vi "Configuration Window.vi"(8 "error in (no error)":errorcluster, 11 "Inst.MOTOR in":refnum<class "Inst.MOTOR.lvclass">) -> (0 "error out":errorcluster, 3 "Inst.MOTOR out":refnum<class "Inst.MOTOR.lvclass">)   [LabVIEW 2019, in "Inst.MOTOR.lvclass"]
uses:
  Inst.MOTOR.lvclass
  Inst.MOTOR.lvclass/Inst.MOTOR.ctl
  <userlib>/LevyLab/Instrument Framework/Instrument Types/VSource/Instrument.VSource.lvclass
panel:
  in  "Termination Character":u8=10 format="%.0x"
  in  "Address":refnum<visa-resource-name>
  in  "flow control":u16(ring) items=["None"=0, "XON/XOFF"=1, "RTS/CTS"=2, "DTR/DSR"=4]
  in  "stop bits":u16(ring)=10 items=["1.0"=10, "1.5"=15, "2.0"=20]
  in  "baud rate":u32(ring)=9600 items=["75"=75, "110"=110, "134"=134, "150"=150, "300"=300, "600"=600, "1200"=1200, "1800"=1800, "2400"=2400, "4800"=4800, "7200"=7200, "9600"=9600, "14400"=14400, "19200"=19200, "28800"=28800, "38400"=38400, "56000"=56000, "57600"=57600, "115200"=115200, "128000"=128000, "230400"=230400]
  in  "parity":enum16{"None", "Odd", "Even", "Mark", "Space"}(ring)
  in  "data bits":u16=8 min=5 max=8 step=1
  in  "Cancel":bool
  in  "OK":bool
  # "confirm or make changes:"
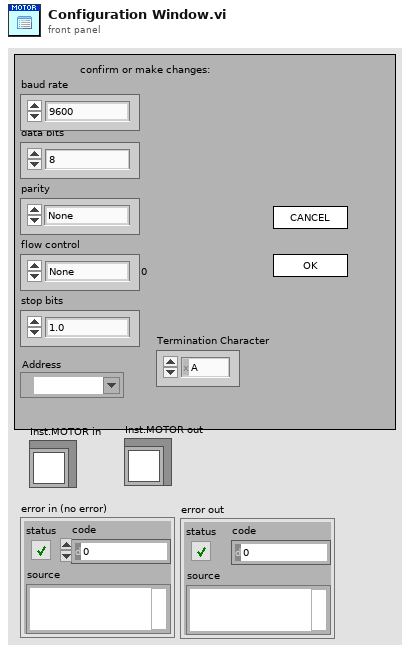
[diagram p1: front panel]
types:
  T1 = enum32{"Invalid", "Standard", "Closed", "Hidden", "Minimized", "Maximized"}
  T2 = enum32{"invalid app kind", "Development System", "Run Time System", "Student Edition", "Embedded LabVIEW", "Evaluation", "Custom"}
  T3 = typedef "Inst.MOTOR.lvclass/Inst.MOTOR.Configuration--Cluster.ctl" = cluster{"baud rate":u32, "data bits":u16, "parity":enum16{"None", "Odd", "Even", "Mark", "Space"}, "stop bits":u16, "flow control":u16, "Read Count":u32, "Address":refnum<visa-resource-name>, "Termination Character":u8}
  T4 = cluster{"Core":cluster{"Current VI Reference":refnum<vi>, "Close Panel on Exit?":bool}, "Configuration":T3}
  T5 = cluster{"Current VI Reference":refnum<vi>, "Close Panel on Exit?":bool}
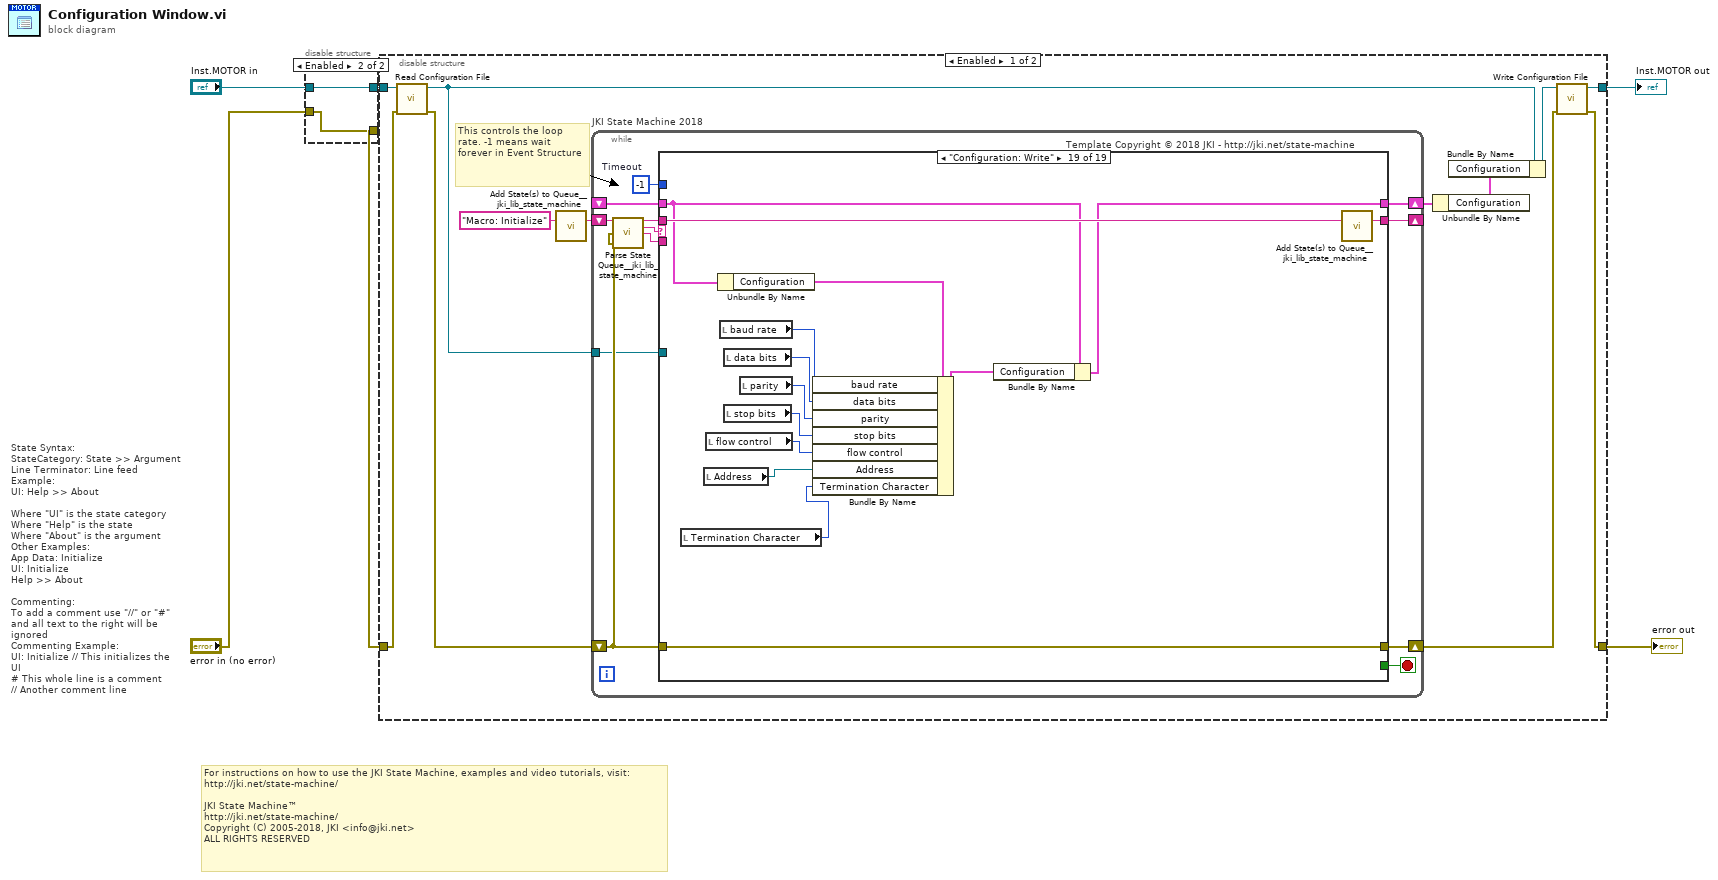
[diagram p0: block diagram]
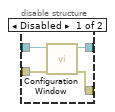
[diagram p2: hidden frame]
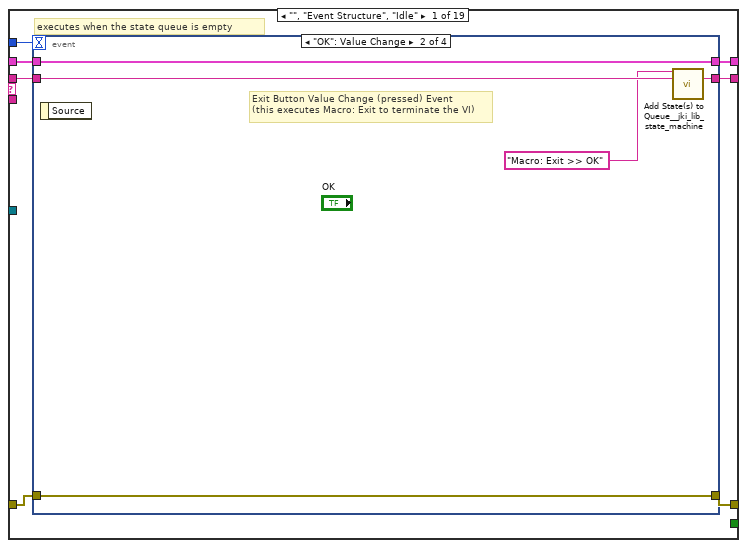
[diagram p3: hidden frame]
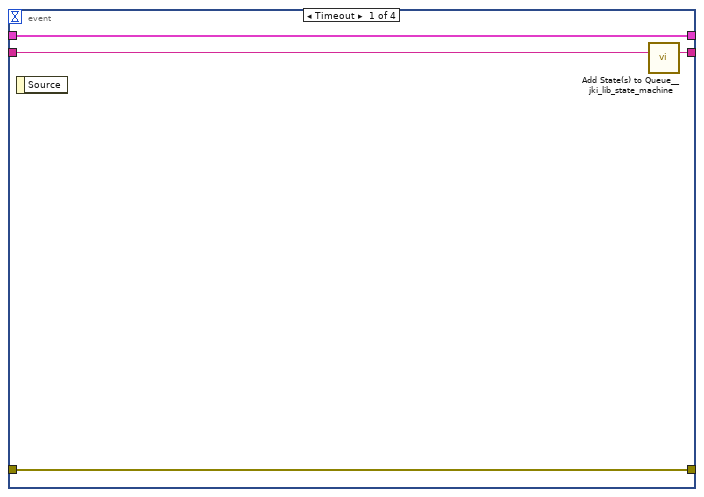
[diagram p4: hidden frame]
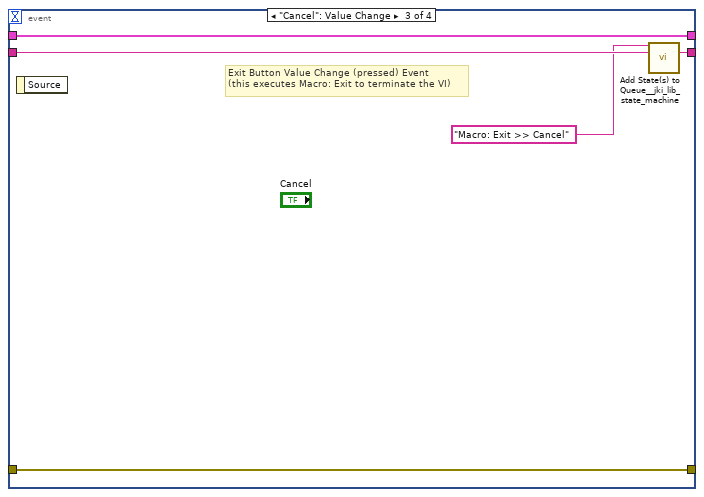
[diagram p5: hidden frame]
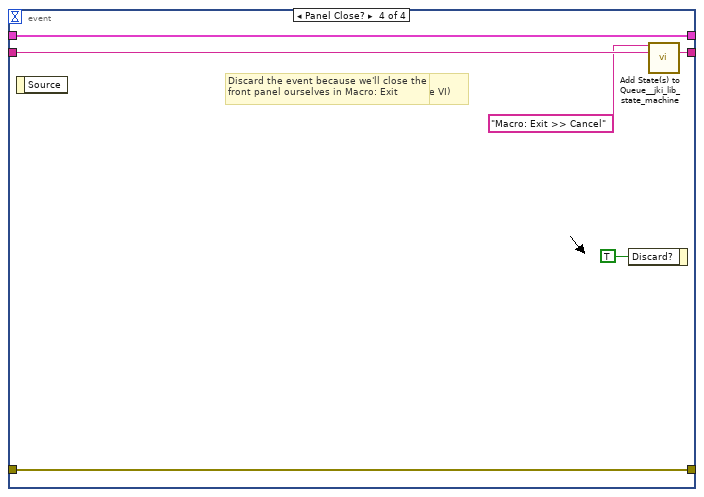
[diagram p6: hidden frame]
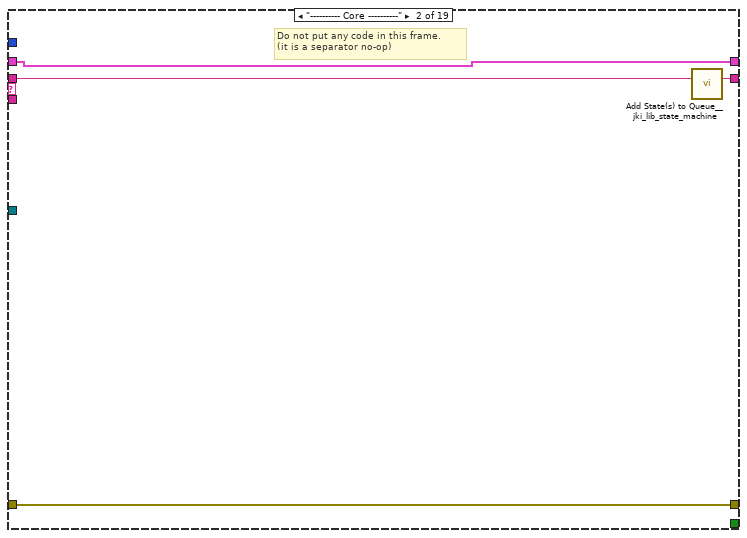
[diagram p7: hidden frame]
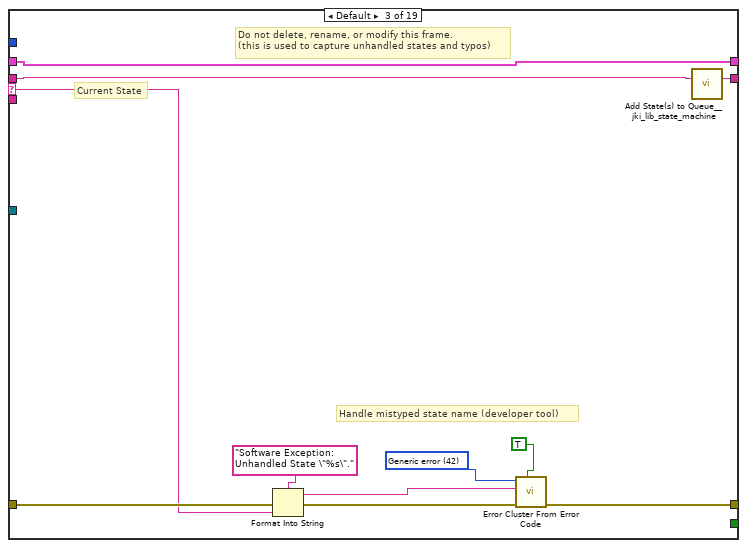
[diagram p8: hidden frame]
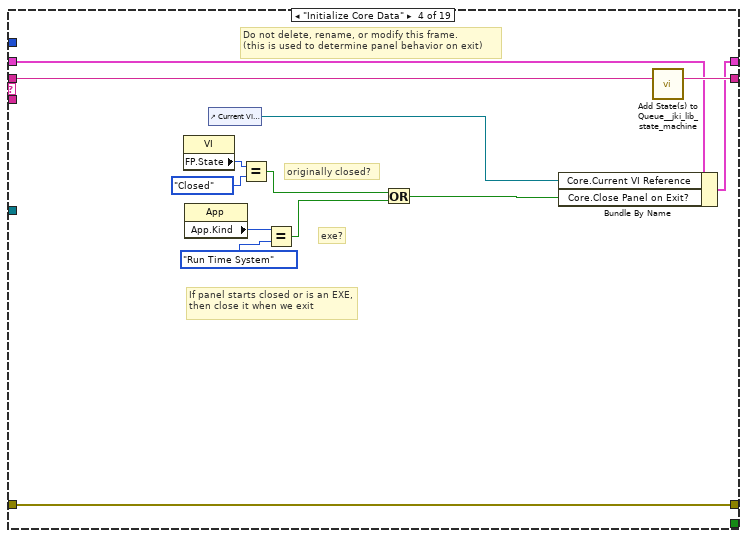
[diagram p9: hidden frame]
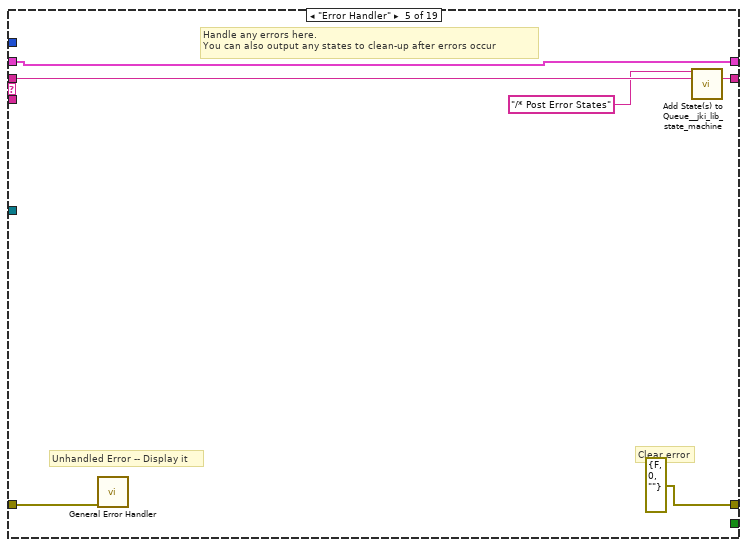
[diagram p10: hidden frame]
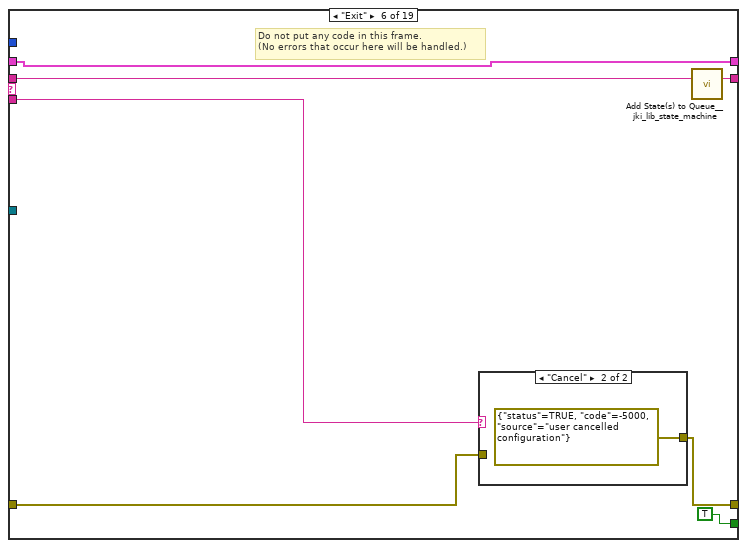
[diagram p11: hidden frame]
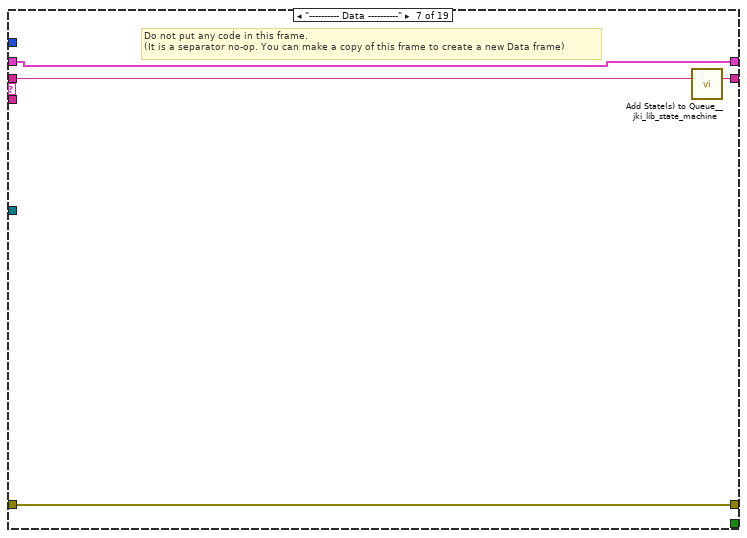
[diagram p13: hidden frame]
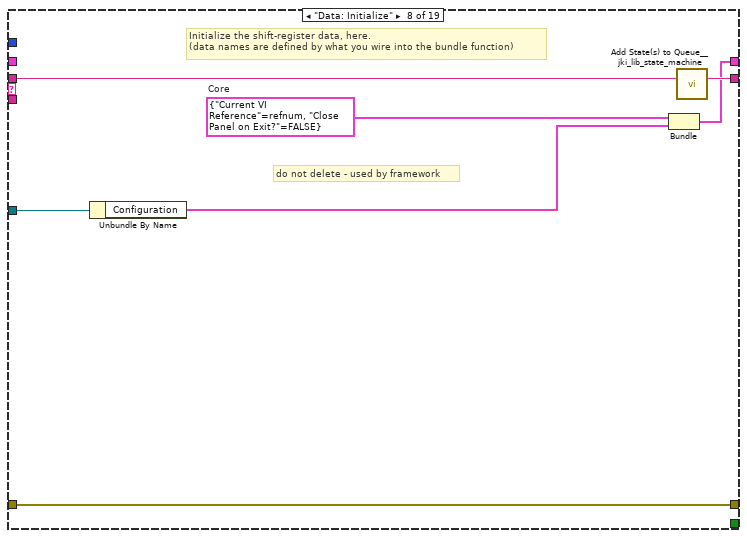
[diagram p14: hidden frame]
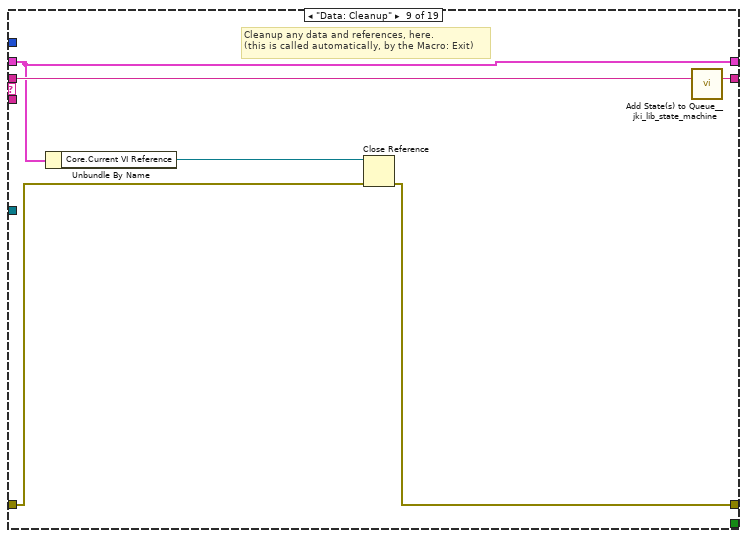
[diagram p15: hidden frame]
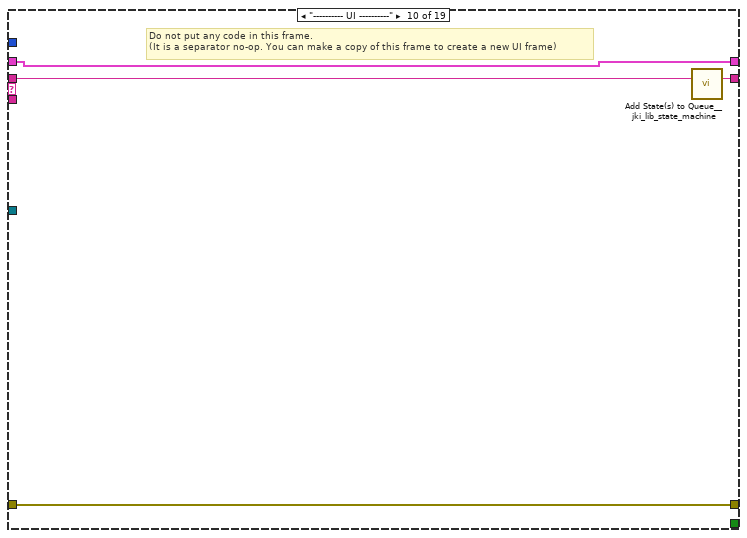
[diagram p16: hidden frame]
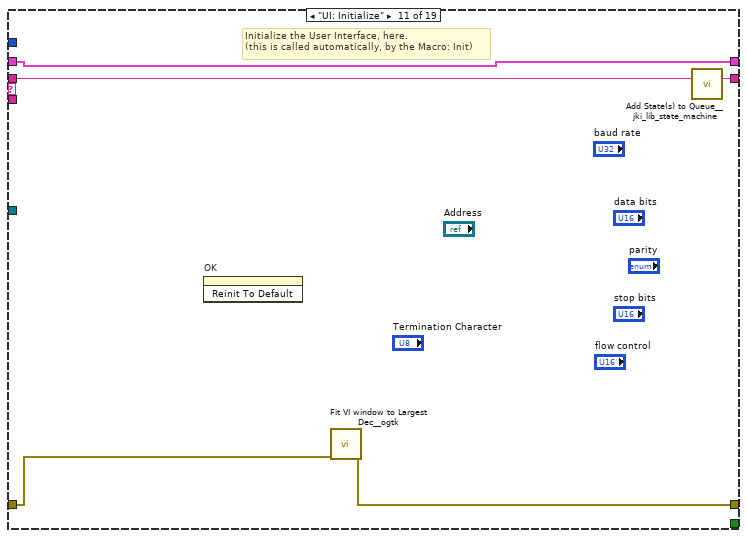
[diagram p17: hidden frame]
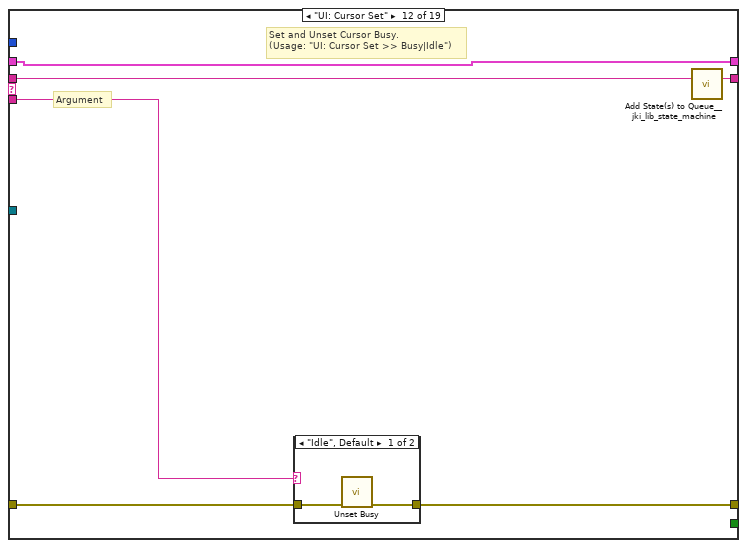
[diagram p18: hidden frame]
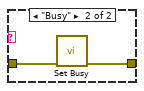
[diagram p19: hidden frame]
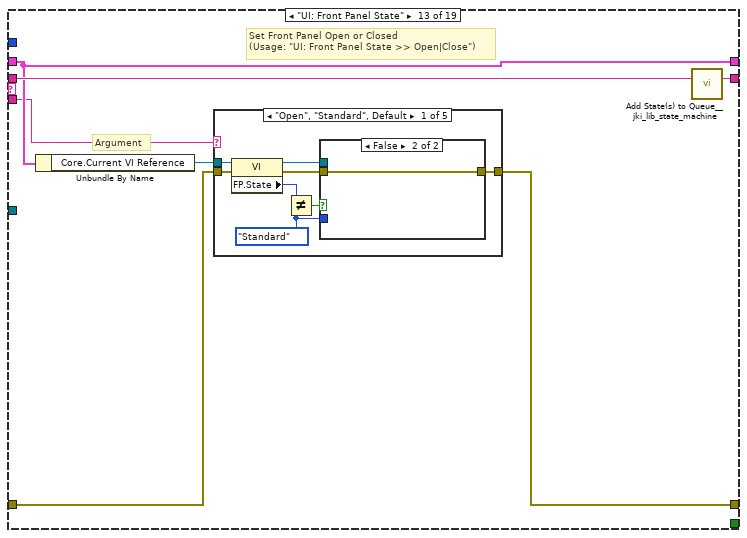
[diagram p20: hidden frame]
diagram:
  # "For instructions on how to use the JKI State Machine, examples and video tutorials, visit:\nhttp://jki.net/state-machine/\n\nJKI State Machine™\nhttp://jki.net/state-machine/\nCopyright (C) 2005-2018, JKI <info@jki.net>\nALL RIGHTS RESERVED"
  # "State Syntax:\nStateCategory: State >> Argument\nLine Terminator: Line feed\nExample:\nUI: Help >> About\n\nWhere \"UI\" is the state category\nWhere \"Help\" is the state\nWhere \"About\" is the argument\nOther Examples:\nApp Data: Initialize\nUI: Initialize\nHelp >> About\n\nCommenting:\nTo add a comment use \"//\" or \"#\" and all text to the right will be ignored\nCommenting Example:\nUI: Initialize // This initializes the UI\n# This whole line is a comment\n// Another comment line"
  n1 = disable-structure shown="Enabled" {
    disable-tunnel: "Inst.MOTOR in" -> [w10 w12]
    disable-tunnel: [w9 w12] -> w3
    disable-tunnel: "error in (no error)" -> [w8 w11]
    disable-tunnel: [w7 w11] -> w1
    frame Disabled {
      n2 = call-parent "Configuration Window.vi"("error in (no error)"=w8, "Instrument"=w10) -> ("error out"=w7:errorcluster, "Instrument out"=w9:refnum<class "Inst.MOTOR.lvclass">)  [unwired: 8 in]
    }
    frame Enabled {
    }
  }
  n3 = disable-structure shown="Enabled" {
    disable-tunnel: [w18 w268] -> w6
    disable-tunnel: [w16 w269] -> w5
    disable-tunnel: w3 -> [w14 w268]
    disable-tunnel: w1 -> [w13 w269]
    frame Enabled {
      # "This controls the loop rate. -1 means wait forever in Event Structure"
      n4 = call-dynamic "Read Configuration File.vi"("error in (no error)"=w13, "Inst.MOTOR in"=w14) -> ("error out"=w15:errorcluster, "Inst.MOTOR out"=w20:refnum<class "Inst.MOTOR.lvclass">)  [unwired: 8 in]
      n5 = call <vilib>:"Add State(s) to Queue__jki_lib_state_machine.vi"("State(s) in (\"\")"="Macro: Initialize") -> ("States Out"=w24:string)  [unwired: 14 in]
      n6 = while "JKI State Machine 2018" {
        shift-right: [w29] -> w22
        shift-left: _ -> [w28]
        shift-right: [w32] -> w17
        shift-left: w15 -> [w26]
        shift-right: [w31] -> _
        shift-left: w24 -> [w33]
        tunnel: w20 -> [w25]
        stop <- w30 stop-if-true
        w27 = -1  # Timeout
        # "Template Copyright © 2018 JKI - http://jki.net/state-machine"
        n7 = call <vilib>:"Parse State Queue__jki_lib_state_machine.vi"("State Queue"=w33, "Error In (no error)"=w26) -> ("Remaining States"=w35:string, "Current State"=w36:string, "Arguments"=w34:string)  [unwired: 11 in]
        n8 = case shown="\"Configuration: Write\"" w36 {
          selector: w36 -> [_ _ w68 _ _ _ _ _ _ _ _ _ _ _ _ _ _ _ _]
          tunnel: w35 -> [w43 w67 w72 w91 w97 w104 w110 w117 w123 w127 w132 w138 w149 w218 w223 w238 w242 w253 w267]
          tunnel: w34 -> [_ _ _ _ _ w100 _ _ _ _ _ w133 w143 _ _ w227 _ _ _]
          tunnel: w28 -> [w41 w64 w70 w84 w94 w102 w107 _ w118 w124 w130 w136 w145 w215 w220 w235 w239 w250 w262]
          tunnel: [w40 w65 w74 w88 errorcluster {"status"=FALSE, "code"=0, "source"=""} ("error out") w98 w108 w113 w119 w125 w128 w134 w146 w216 w221 w236 w240 w251 w265] -> w32
          tunnel: w26 -> [w39 w65 w73 w88 w93 w99 w108 w113 w120 w125 w129 w135 w147 w216 w221 w236 w240 w251 w265]
          tunnel: [w42 w66 w71 w90 w96 w103 w109 w116 w122 w126 w131 w137 w148 w217 w222 w237 w241 w252 w266] -> w31
          tunnel: [_ _ _ _ _ TRUE _ _ _ _ _ _ _ _ _ _ _ _ _] -> w30
          tunnel: [w38 w64 w70 w89 w94 w102 w107 w115 w118 w124 w130 w136 w145 w215 w220 w235 w239 w250 w261] -> w29
          tunnel: w27 -> [w37 _ _ _ _ _ _ _ _ _ _ _ _ _ _ _ _ _ _]
          tunnel: w25 -> [_ _ _ _ _ _ _ w112 _ _ _ _ _ _ _ _ _ _ _]
          frame "", "Event Structure", "Idle" {
            # "executes when the state queue is empty"
            n9 = event shown="[1] \"OK\": Value Change" {
              selector: _ -> [_ _ _ _]
              dyn-events: _ -> [_ _ _ _]
              timeout: w37 -> [_ _ _ _]
              tunnel: w43 -> [w47 w52 w57 w63]
              tunnel: [w46 w51 w56 w62] -> w42
              tunnel: w41 -> [w44 w49 w54 w60]
              tunnel: [w45 w50 w55 w61] -> w40
              tunnel: w39 -> [w45 w50 w55 w61]
              tunnel: [w44 w49 w54 w60] -> w38
              event Timeout {
                n10 = event-data() -> ()  [unwired: 1 in, 1 out]
                n11 = call <vilib>:"Add State(s) to Queue__jki_lib_state_machine.vi"("State(s) in (\"\")"=w47) -> ("States Out"=w46:string)  [unwired: 14 in]
              }
              event "OK": Value Change {
                # "Exit Button Value Change (pressed) Event\n(this executes Macro: Exit to terminate the VI)"
                n12 = event-data() -> ()  [unwired: 1 in, 1 out]
                n13 = call <vilib>:"Add State(s) to Queue__jki_lib_state_machine.vi"("State(s) in Front (\"\")"="Macro: Exit >> OK", "State(s) in (\"\")"=w52) -> ("States Out"=w51:string)  [unwired: 13 in]
              }
              event "Cancel": Value Change {
                # "Exit Button Value Change (pressed) Event\n(this executes Macro: Exit to terminate the VI)"
                n14 = event-data() -> ()  [unwired: 1 in, 1 out]
                n15 = call <vilib>:"Add State(s) to Queue__jki_lib_state_machine.vi"("State(s) in Front (\"\")"="Macro: Exit >> Cancel", "State(s) in (\"\")"=w57) -> ("States Out"=w56:string)  [unwired: 13 in]
              }
              event Panel Close? {
                # "Discard the event because we'll close the front panel ourselves in Macro: Exit"
                # "Close Panel button (pressed) Event\n(this executes Macro: Exit to terminate the VI)"
                n16 = event-data() -> ()  [unwired: 1 in, 1 out]
                n17 = event-data("Discard?"=TRUE) -> ()  [unwired: 1 in, 1 out]
                n18 = call <vilib>:"Add State(s) to Queue__jki_lib_state_machine.vi"("State(s) in Front (\"\")"="Macro: Exit >> Cancel", "State(s) in (\"\")"=w63) -> ("States Out"=w62:string)  [unwired: 13 in]
              }
            }
          }
          frame "---------- Core ----------" {
            # "Do not put any code in this frame.\n(it is a separator no-op)"
            n19 = call <vilib>:"Add State(s) to Queue__jki_lib_state_machine.vi"("State(s) in (\"\")"=w67) -> ("States Out"=w66:string)  [unwired: 14 in]
          }
          frame Default {
            w77 = 42 items=["No error", "Argument error", "Memory is full", "Out of zone", "End of file", "File already open", "Generic file I/O error", "File not found", "File permission error", "Disk is full", "Duplicate path", "Too many files open", "System feature not enabled", "Resource file not found", "Cannot add resource", "Resource not found", "Image not found", "Image memory error", "Pen does not exist", "Config type invalid", "Config token not found", "Config parse error", "Config memory error", "Bad external code format", "Bad external code offset", "External code not present", "Null window", "Destroy window error", "Null menu", "Print aborted", "Bad print record", "Print driver error", "Windows error during printing", "Memory error during printing", "Print dialog error", "Generic print error", "Invalid device refnum", "Device not found", "Device parameter error", "Device unit error", "Cannot open device", "Device call aborted", "Generic error", "Cancelled by user", "Object ID too low", "Object ID too high", "Object not in heap", "Unknown heap", "Unknown object (invalid DefProc)", "Unknown object (DefProc not in table)", "Message out of range", "Invalid (null) method", "Unknown message", "Manager call not supported", "Bad address", "Network operation in progress", "Network operation timed out", "Connection is busy", "Network attribute not supported", "Network error", "Address in use", "System out of memory", "Connection aborted", "Connection refused", "Not connected", "Already connected", "Connection closed", "Initialization error (interapplication manager)", "Bad occurrence", "Wait on unbound occurrence handler", "Occurrence queue overflow", "Datalog type conflict", "Unused", "Unrecognized type (interapplication manager)", "Memory corrupt", "Failed to make temporary DLL", "Old CIN version", "Drag socket not found", "Failed to load drop-object", "Failed to register OLE object", "Failed to release OLE object", "Format specifier type mismatch", "Unknown format specifier", "Too few format specifiers", "Too many format specifiers", "Scan failed", "Newer CIN version", "Error converting to variant", "Runtime menu error", "Password tampered", "Variant attribute not found", "Incompatible variant data type", "Event data is not available", "Event Store is not present", "Occurrence is not found", "Event Queue is not created", "Event info is not available", "Refnum passed is NULL", "Error retrieving Class GUID", "Error retrieving CoClass GUID", "Error retrieving TypeLib GUID.", "Bad built application magic bytes.", "Specific driver is different from the specific driver associated with the Logical Name.", "There is no session opened to the class driver.", "Max Error", "MAX - Error with config objects", "MAX - Error loading configuration", "MAX - Group not supported"]
            # "Current State"
            # "Do not delete, rename, or modify this frame.\n(this is used to capture unhandled states and typos)"
            # "Handle mistyped state name (developer tool)"
            n20 = Format Into String(format string="Software Exception: Unhandled State \"%s\"." ("message"), error in=w73, w68) -> (resulting string=w76:string, error out=w75:errorcluster)  [unwired: 1 in]
            n21 = call <vilib>:"Error Cluster From Error Code.vi"("show call chain? (False)"=TRUE, "error in (no error)"=w75, "error message (\"\")"=w76, "error code (0)"=w77) -> ("error out"=w74:errorcluster)  [unwired: 5 in]
            n22 = call <vilib>:"Add State(s) to Queue__jki_lib_state_machine.vi"("State(s) in (\"\")"=w72) -> ("States Out"=w71:string)  [unwired: 14 in]
          }
          frame "Initialize Core Data" {
            # "Do not delete, rename, or modify this frame.\n(this is used to determine panel behavior on exit)"
            # "originally closed?"
            # "exe?"
            # "If panel starts closed or is an EXE, then close it when we exit"
            n23 = property class="VI"() -> ("FP.State"=w81:T1)  [unwired: 2 in, 2 out]
            n24 = property class="App"() -> ("App.Kind"=w87:T2)  [unwired: 2 in, 2 out]
            n25 = control-ref of="Current VI Reference"() -> (w82:refnum<vi>)
            n26 = Equal?(x=w81, y=T1."Closed" ("Front Panel Window:State")) -> (x = y?=w79:bool)
            n27 = Equal?(x=w87, y=T2."Run Time System" ("Application:Kind")) -> (x = y?=w85:bool)
            n28 = Or(x=w79, y=w85) -> (x .or. y?=w83:bool)
            n29 = Bundle By Name(cluster=w84, "Core.Current VI Reference"=w82, "Core.Close Panel on Exit?"=w83) -> (w89:T4)
            n30 = call <vilib>:"Add State(s) to Queue__jki_lib_state_machine.vi"("State(s) in (\"\")"=w91) -> ("States Out"=w90:string)  [unwired: 14 in]
          }
          frame "Error Handler" {
            # "Unhandled Error -- Display it"
            # "Handle any errors here.\nYou can also output any states to clean-up after errors occur"
            # "Clear error"
            n31 = call <vilib>:"General Error Handler.vi"("error in (no error)"=w93) -> ()  [unwired: 10 in, 5 out]
            n32 = call <vilib>:"Add State(s) to Queue__jki_lib_state_machine.vi"("State(s) in Front (\"\")"="/* Post Error States", "State(s) in (\"\")"=w97) -> ("States Out"=w96:string)  [unwired: 13 in]
          }
          frame "Exit" {
            # "Do not put any code in this frame.\n(No errors that occur here will be handled.)"
            n33 = case shown="\"Cancel\"" w100 {
              tunnel: w99 -> [w105 _]
              tunnel: [w105 errorcluster {"status"=TRUE, "code"=-5000, "source"="user cancelled configuration"} ("error in (no error)")] -> w98
              frame "OK", Default {
              }
              frame "Cancel" {
              }
            }
            n34 = call <vilib>:"Add State(s) to Queue__jki_lib_state_machine.vi"("State(s) in (\"\")"=w104) -> ("States Out"=w103:string)  [unwired: 14 in]
          }
          frame "---------- Data ----------" {
            # "Do not put any code in this frame.\n(It is a separator no-op. You can make a copy of this frame to create a new Data frame)"
            n35 = call <vilib>:"Add State(s) to Queue__jki_lib_state_machine.vi"("State(s) in (\"\")"=w110) -> ("States Out"=w109:string)  [unwired: 14 in]
          }
          frame "Data: Initialize" {
            w114 = T5 {"Current VI Reference"=refnum, "Close Panel on Exit?"=FALSE}  # Core
            # "do not delete - used by framework"
            # "Initialize the shift-register data, here.\n(data names are defined by what you wire into the bundle function)"
            n36 = Unbundle By Name(w112) -> ("Configuration"=w111:T3)
            n37 = Bundle("Core"=w114, "Configuration"=w111) -> (w115:T4)  [unwired: 1 in]
            n38 = call <vilib>:"Add State(s) to Queue__jki_lib_state_machine.vi"("State(s) in (\"\")"=w117) -> ("States Out"=w116:string)  [unwired: 14 in]
          }
          frame "Data: Cleanup" {
            # "Cleanup any data and references, here.\n(this is called automatically, by the Macro: Exit)"
            n39 = Unbundle By Name(w118) -> ("Core.Current VI Reference"=w121:refnum<vi>)
            n40 = Close Reference(reference=w121, error in (no error)=w120) -> (error out=w119:errorcluster)
            n41 = call <vilib>:"Add State(s) to Queue__jki_lib_state_machine.vi"("State(s) in (\"\")"=w123) -> ("States Out"=w122:string)  [unwired: 14 in]
          }
          frame "---------- UI ----------" {
            # "Do not put any code in this frame.\n(It is a separator no-op. You can make a copy of this frame to create a new UI frame)"
            n42 = call <vilib>:"Add State(s) to Queue__jki_lib_state_machine.vi"("State(s) in (\"\")"=w127) -> ("States Out"=w126:string)  [unwired: 14 in]
          }
          frame "UI: Initialize" {
            # "Initialize the User Interface, here.\n(this is called automatically, by the Macro: Init)"
            n43 = invoke on="OK" class="Bool" method="Reinit To Default"() -> ()  [unwired: 3 in, 3 out]
            n44 = call <userlib>:"Fit VI window to Largest Dec__ogtk.vi"("error in (no error)"=w129) -> ("error out"=w128:errorcluster)  [unwired: 5 in, 1 out]
            n45 = call <vilib>:"Add State(s) to Queue__jki_lib_state_machine.vi"("State(s) in (\"\")"=w132) -> ("States Out"=w131:string)  [unwired: 14 in]
          }
          frame "UI: Cursor Set" {
            # "Argument"
            # "Set and Unset Cursor Busy.\n(Usage: \"UI: Cursor Set >> Busy|Idle\")"
            n46 = case shown="\"Idle\", Default" w133 {
              tunnel: w135 -> [w140 w142]
              tunnel: [w139 w141] -> w134
              frame "Idle", Default {
                n47 = call <vilib>:"Unset Busy.vi"("error in (no error)"=w140) -> ("error out"=w139:errorcluster)  [unwired: 10 in]
              }
              frame "Busy" {
                n48 = call <vilib>:"Set Busy.vi"("error in (no error)"=w142) -> ("error out"=w141:errorcluster)  [unwired: 9 in, 1 out]
              }
            }
            n49 = call <vilib>:"Add State(s) to Queue__jki_lib_state_machine.vi"("State(s) in (\"\")"=w138) -> ("States Out"=w137:string)  [unwired: 14 in]
          }
          frame "UI: Front Panel State" {
            # "Argument"
            # "Set Front Panel Open or Closed\n(Usage: \"UI: Front Panel State >> Open|Close\")"
            n50 = Unbundle By Name(w145) -> ("Core.Current VI Reference"=w144:refnum<vi>)
            n51 = case shown="\"Open\", \"Standard\", Default" w143 {
              tunnel: w147 -> [w155 w170 w181 w194 w207]
              tunnel: [w157 w171 w183 w196 w209] -> w146
              tunnel: w144 -> [w156 w168 w182 w195 w208]
              frame "Open", "Standard", Default {
                w150 = T1."Standard" ("State")
                n52 = property class="VI"(reference=w156, error in=w155) -> (reference out=w153:refnum<vi>, error out=w154:errorcluster, "FP.State"=w152:T1)
                n53 = Not Equal?(x=w152, y=w150) -> (x != y?=w151:bool)
                n54 = case shown="False" w151 {
                  tunnel: [w161 w163] -> w157
                  tunnel: w154 -> [w160 w163]
                  tunnel: w153 -> [w159 _]
                  tunnel: w150 -> [w158 _]
                  frame True {
                    n55 = invoke class="VI" method="FP.Open"(reference=w159, error in=w160, "Activate"=TRUE, "State"=w158) -> (error out=w161:errorcluster)  [unwired: 1 in, 4 out]
                  }
                  frame False {
                  }
                }
              }
              frame "Close", "Closed" {
                n56 = property class="VI"(reference=w168, error in=w170) -> (reference out=w167:refnum<vi>, error out=w169:errorcluster, "FP.State"=w165:T1)
                n57 = Not Equal?(x=w165, y=T1."Closed" ("Front Panel Window:State")) -> (x != y?=w164:bool)
                n58 = case shown="True" w164 {
                  tunnel: [w172 w175] -> w171
                  tunnel: w169 -> [w172 w174]
                  tunnel: w167 -> [_ w173]
                  frame False {
                  }
                  frame True {
                    n59 = invoke class="VI" method="FP.Close"(reference=w173, error in=w174) -> (error out=w175:errorcluster)  [unwired: 1 in, 2 out]
                  }
                }
              }
              frame "Hidden", "Hide" {
                w176 = T1."Hidden" ("State")
                n60 = property class="VI"(reference=w182, error in=w181) -> (reference out=w179:refnum<vi>, error out=w180:errorcluster, "FP.State"=w178:T1)
                n61 = Not Equal?(x=w178, y=w176) -> (x != y?=w177:bool)
                n62 = case shown="True" w177 {
                  tunnel: [w187 w188] -> w183
                  tunnel: w180 -> [w186 w188]
                  tunnel: w179 -> [w185 _]
                  tunnel: w176 -> [w184 _]
                  frame True {
                    n63 = invoke class="VI" method="FP.Open"(reference=w185, error in=w186, "State"=w184) -> (error out=w187:errorcluster)  [unwired: 2 in, 4 out]
                  }
                  frame False {
                  }
                }
              }
              frame "Minimize", "Minimized" {
                w189 = T1."Minimized" ("State")
                n64 = property class="VI"(reference=w195, error in=w194) -> (reference out=w192:refnum<vi>, error out=w193:errorcluster, "FP.State"=w191:T1)
                n65 = Not Equal?(x=w191, y=w189) -> (x != y?=w190:bool)
                n66 = case shown="True" w190 {
                  tunnel: [w200 w201] -> w196
                  tunnel: w193 -> [w199 w201]
                  tunnel: w192 -> [w198 _]
                  tunnel: w189 -> [w197 _]
                  frame True {
                    n67 = invoke class="VI" method="FP.Open"(reference=w198, error in=w199, "State"=w197) -> (error out=w200:errorcluster)  [unwired: 2 in, 4 out]
                  }
                  frame False {
                  }
                }
              }
              frame "Maximize", "Maximized" {
                w202 = T1."Maximized" ("State")
                n68 = property class="VI"(reference=w208, error in=w207) -> (reference out=w205:refnum<vi>, error out=w206:errorcluster, "FP.State"=w204:T1)
                n69 = Not Equal?(x=w204, y=w202) -> (x != y?=w203:bool)
                n70 = case shown="True" w203 {
                  tunnel: [w213 w214] -> w209
                  tunnel: w206 -> [w212 w214]
                  tunnel: w205 -> [w211 _]
                  tunnel: w202 -> [w210 _]
                  frame True {
                    n71 = invoke class="VI" method="FP.Open"(reference=w211, error in=w212, "State"=w210) -> (error out=w213:errorcluster)  [unwired: 2 in, 4 out]
                  }
                  frame False {
                  }
                }
              }
            }
            n72 = call <vilib>:"Add State(s) to Queue__jki_lib_state_machine.vi"("State(s) in (\"\")"=w149) -> ("States Out"=w148:string)  [unwired: 14 in]
          }
          frame "---------- Macro ----------" {
            # "Do not put any code in this frame.\n(It is a separator no-op. You can make a copy of this frame to create a new Macro frame)"
            n73 = call <vilib>:"Add State(s) to Queue__jki_lib_state_machine.vi"("State(s) in (\"\")"=w218) -> ("States Out"=w217:string)  [unwired: 14 in]
          }
          frame "Macro: Initialize" {
            w219 = "Data: Initialize\nInitialize Core Data\nUI: Initialize\nUI: Front Panel State >> Open\nConfiguration: Read"  # Data: Initialize Initialize Core Data UI: Initialize UI: Front Panel State >> Open Configuration: Read
            # "Initialization Macro\n(This is called once, when the VI starts)"
            n74 = call <vilib>:"Add State(s) to Queue__jki_lib_state_machine.vi"("State(s) in Front (\"\")"=w219, "State(s) in (\"\")"=w223) -> ("States Out"=w222:string)  [unwired: 13 in]
          }
          frame "Macro: Exit" {
            # "Exit Macro\n(This is called once, when the VI exits)"
            n75 = Unbundle By Name(w235) -> ("Core.Close Panel on Exit?"=w234:bool)
            n76 = call <vilib>:"Build State String with Arguments__JKI_lib_State_Machine.vi"("Arguments (\"\")"=w227, "State"="Exit") -> ("State with Arguments"=w225:string)  [unwired: 4 in]
            n77 = Select(t="UI: Front Panel State >> Close", s=w234, f="" ("Empty String Constant")) -> (s? t:f=w231:string)
            n78 = call <vilib>:"Add State(s) to Queue__jki_lib_state_machine.vi"("State(s) in Front (\"\")"="Data: Cleanup", "State(s) at Back (\"\")"=w225) -> ("States Out"=w224:string)  [unwired: 13 in]
            n79 = call <vilib>:"Add State(s) to Queue__jki_lib_state_machine.vi"("State(s) in Front (\"\")"="Configuration: Write", "State(s) in (\"\")"=w231, "State(s) at Back (\"\")"=w224) -> ("States Out"=w230:string)  [unwired: 12 in]
            n80 = call <vilib>:"Add State(s) to Queue__jki_lib_state_machine.vi"("State(s) in Front (\"\")"=w230, "State(s) in (\"\")"=w238) -> ("States Out"=w237:string)  [unwired: 13 in]
          }
          frame "---------- Configuration ----------" {
            # "Template Separator\n(You can make a copy of, or modify, this frame)"
            n81 = call <vilib>:"Add State(s) to Queue__jki_lib_state_machine.vi"("State(s) in (\"\")"=w242) -> ("States Out"=w241:string)  [unwired: 14 in]
          }
          frame "Configuration: Read" {
            # "Your code here.\n(You can make a copy of, or modify, this frame)"
            n82 = Unbundle By Name(w250) -> ("Configuration"=w249:T3)
            n83 = Unbundle By Name(w249) -> ("baud rate"=w248:u32, "data bits"=w247:u16, "parity"=w246:enum16{"None", "Odd", "Even", "Mark", "Space"}, "stop bits"=w245:u16, "flow control"=w244:u16, "Termination Character"=w243:u8)
            n84 = local write "Termination Character"(w243) -> ()
            n85 = local write "flow control"(w244) -> ()
            n86 = local write "stop bits"(w245) -> ()
            n87 = local write "baud rate"(w248) -> ()
            n88 = local write "parity"(w246) -> ()
            n89 = local write "data bits"(w247) -> ()
            n90 = call <vilib>:"Add State(s) to Queue__jki_lib_state_machine.vi"("State(s) in (\"\")"=w253) -> ("States Out"=w252:string)  [unwired: 14 in]
          }
          frame "Configuration: Write" {
            n91 = local read "Termination Character"() -> (w254:u8)
            n92 = local read "Address"() -> (w255:refnum<visa-resource-name>)
            n93 = local read "flow control"() -> (w256:u16)
            n94 = Unbundle By Name(w262) -> ("Configuration"=w264:T3)
            n95 = local read "baud rate"() -> (w260:u32)
            n96 = local read "data bits"() -> (w259:u16)
            n97 = local read "stop bits"() -> (w257:u16)
            n98 = local read "parity"() -> (w258:enum16{"None", "Odd", "Even", "Mark", "Space"})
            n99 = Bundle By Name(cluster=w264, "baud rate"=w260, "data bits"=w259, "parity"=w258, "stop bits"=w257, "flow control"=w256, "Address"=w255, "Termination Character"=w254) -> (w263:T3)
            n100 = Bundle By Name(cluster=w262, "Configuration"=w263) -> (w261:T4)
            n101 = call <vilib>:"Add State(s) to Queue__jki_lib_state_machine.vi"("State(s) in (\"\")"=w267) -> ("States Out"=w266:string)  [unwired: 14 in]
          }
        }
      }
      n102 = Unbundle By Name(w22) -> ("Configuration"=w21:T3)
      n103 = Bundle By Name(cluster=w20, "Configuration"=w21) -> (w19:refnum<class "Inst.MOTOR.lvclass">)
      n104 = call-dynamic "Write Configuration File.vi"("error in (no error)"=w17, "Inst.MOTOR in"=w19) -> ("error out"=w16:errorcluster, "Inst.MOTOR out"=w18:refnum<class "Inst.MOTOR.lvclass">)  [unwired: 8 in]
    }
    frame Disabled {
    }
  }
  "error out" <- w5
  "Inst.MOTOR out" <- w6
